vi "GetPublishedTopics.vi"(8 "Status":T4[](array[typedef]), 10 "servers":T3[](array[typedef])) -> (1 "Topic Types":string[](array[string]), 3 "Published Topics":string[](array[string]))   [LabVIEW 2012]
doc: "Gets all topics that are published by this node."
uses:
  <userlib>/ROSforLV/ROS/Code/Console/Servers/ServerSubs/MyState.ctl
  <userlib>/ROSforLV/ROS/Code/Console/Servers/ServerSubs/ServoInfo.ctl
  <userlib>/ROSforLV/ROS/Code/SubVIs/_ROSControl.ctl
  <userlib>/ROSforLV/ROS/Code/SubVIs/_ROSDirection.ctl
panel:
  in  "Node ROS":T1={"topic port"=0, "Node"="", "topic"="", "type"="", "node port"=0, "error "={"status"=FALSE, "code"=0, "source"=""}, "Direction"=enum."Node", "APIs"=[], "Update (ms)"=1, "write queue"=1}
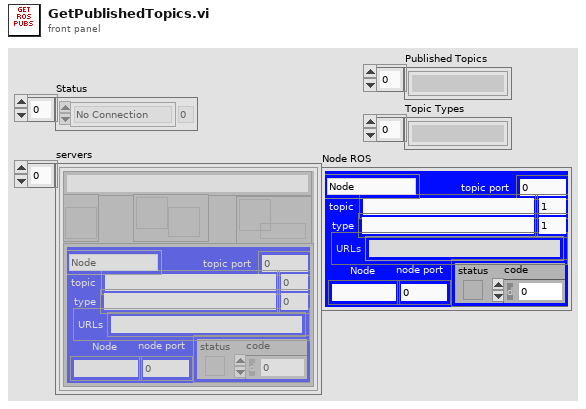
[diagram p1: front panel]
types:
  T1 = typedef "_ROSControl.ctl" = cluster{"topic port":u16, "Node":string, "topic":string, "type":string, "node port":u32, "error ":errorcluster, "Direction":T2, "APIs":string[], "Update (ms)":u16, "write queue":u16}
  T2 = typedef "_ROSDirection.ctl" = enum16{"Node", "Publisher", "Subscriber", "Service Client"}
  T3 = typedef "ServoInfo.ctl" = cluster{"vi name":string, "VI Refnum":refnum<vi>, "queue":refnum<queue>, "ROS":T1, "notifier":refnum<notifier>}
  T4 = typedef "MyState.ctl" = enum16{"No Connection", "Registered", "Connected", "Close"}
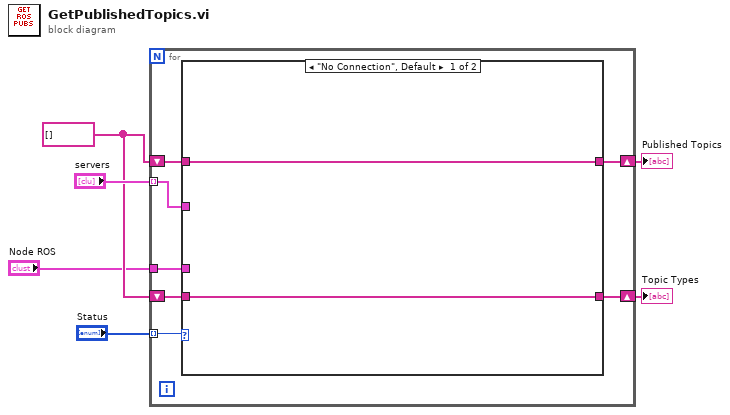
[diagram p0: block diagram]
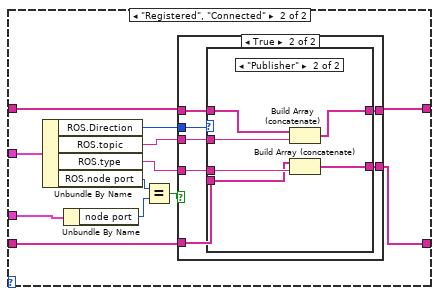
[diagram p2: hidden frame]
diagram:
  w3 = string[] []
  n1 = for {
    tunnel: "servers" -> [w13] mode=indexing
    tunnel: "Status" -> [w7] mode=indexing
    shift-right: [w12] -> w4
    shift-left: w3 -> [w11]
    shift-right: [w10] -> w2
    shift-left: w3 -> [w9]
    tunnel: "Node ROS" -> [w8]
    n2 = case shown="\"No Connection\", Default" w7 {
      tunnel: w13 -> [_ w27]
      tunnel: [w15 w25] -> w12
      tunnel: w11 -> [w15 w24]
      tunnel: [w14 w21] -> w10
      tunnel: w9 -> [w14 w20]
      tunnel: w8 -> [_ w19]
      frame "No Connection", Default {
      }
      frame "Registered", "Connected" {
        n3 = Unbundle By Name(w27) -> ("ROS.Direction"=w23:T2, "ROS.topic"=w26:string, "ROS.type"=w22:string, "ROS.node port"=w17:u32)
        n4 = Unbundle By Name(w19) -> ("node port"=w16:u32)
        n5 = Equal?(x=w17, y=w16) -> (x = y?=w18:bool)
        n6 = case shown="True" w18 {
          tunnel: w26 -> [_ w36]
          tunnel: [w29 w35] -> w25
          tunnel: w24 -> [w29 w34]
          tunnel: w23 -> [_ w33]
          tunnel: w22 -> [_ w32]
          tunnel: [w28 w31] -> w21
          tunnel: w20 -> [w28 w30]
          frame False {
          }
          frame True {
            n7 = case shown="\"Publisher\"" w33 {
              tunnel: w36 -> [_ w44]
              tunnel: [w38 w42] -> w35
              tunnel: w34 -> [w38 w43]
              tunnel: w32 -> [_ w41]
              tunnel: [w37 w40] -> w31
              tunnel: w30 -> [w37 w39]
              frame "Node", Default {
              }
              frame "Publisher" {
                n8 = Build Array (concatenate)(w43, w44) -> (w42:string[])
                n9 = Build Array (concatenate)(w39, w41) -> (w40:string[])
              }
            }
          }
        }
      }
    }
  }
  "Published Topics" <- w4
  "Topic Types" <- w2
